vi "Resource Type.vi"(8 "error in (no error)":errorcluster, 11 "DeployTcpResource in":refnum<class "TcpResource.lvclass">) -> (0 "error out":errorcluster, 2 "Resource Type":string, 3 "DeployTcpResource out":refnum<class "TcpResource.lvclass">)   [LabVIEW 2020, in "PicoG-Core.lvlib" / "TcpResource.lvclass"]
uses:
  TcpResource.lvclass
  TcpResource.lvclass/TcpResource.ctl
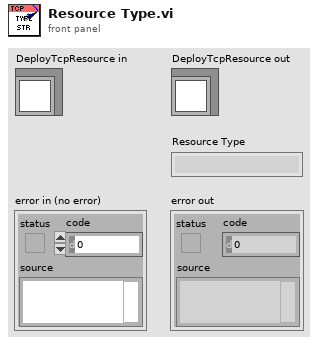
[diagram p1: front panel]
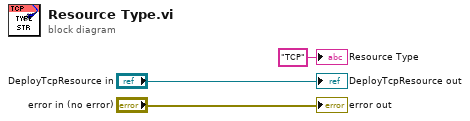
[diagram p0: block diagram]
diagram:
  "error out" <- "error in (no error)"
  "DeployTcpResource out" <- "DeployTcpResource in"
  "Resource Type" <- "TCP" ("Resource Type")
